vi "Verify Can Add Additional Bitfile.vi"(8 "error in (no error)":errorcluster, 10 "RIO Device Addresses":string[](array[string]), 11 "Item Ref in":T1 format="%.0x") -> (0 "error out":errorcluster, 2 "Can Add?":bool, 3 "Item Ref out":T1 format="%.0x")   [LabVIEW 2015, in "Engine Simulation Toolkit System Explorer.lvlib"]
uses:
  Engine Simulation Toolkit System Explorer.lvlib
  <vilib>/NI Veristand/Custom Device API/Custom Device Item Ref.ctl
  Shared/Bitfile EST Version.ctl
  Shared/Properties.vi
  <vilib>/NI Veristand/Custom Device API/Get Item Property (String).vi
  Shared/Engine Simulation Toolkit Shared.lvlib
  <vilib>/NI VeriStand/Custom Device API/Custom Device API.lvlib
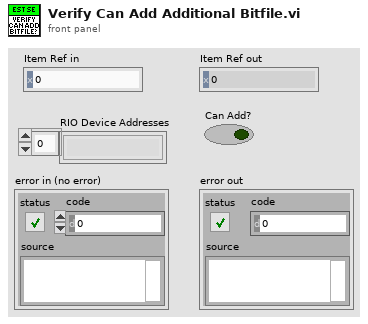
[diagram p1: front panel]
types:
  T1 = typedef "Custom Device API.lvlib/Custom Device Item Ref.ctl" = u64
  T2 = typedef "Engine Simulation Toolkit Shared.lvlib/Bitfile EST Version.ctl" = enum16{"1.0", "1.1", "1.2", "1.3", "1.4"}
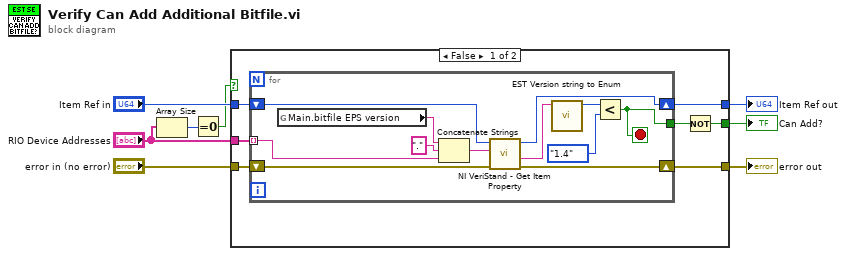
[diagram p0: block diagram]
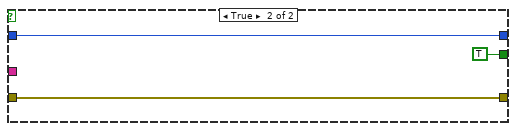
[diagram p2: hidden frame]
diagram:
  n1 = Array Size(array="RIO Device Addresses") -> (size(s)=w2:i32)
  n2 = Equal To 0?(x=w2) -> (x = 0?=w1:bool)
  n3 = case shown="False" w1 {
    tunnel: [w14 w28] -> w8
    tunnel: "Item Ref in" -> [w13 w28]
    tunnel: [w12 w29] -> w6
    tunnel: "error in (no error)" -> [w11 w29]
    tunnel: [w10 TRUE] -> w4
    tunnel: "RIO Device Addresses" -> [w9 _]
    frame False {
      n4 = for {
        tunnel: w9 -> [w25] mode=indexing
        shift-right: [w23] -> w12
        shift-left: w11 -> [w24]
        shift-right: [w20] -> w14
        shift-left: w13 -> [w21]
        tunnel: [w16] -> w15
        stop <- w16 stop-if-true
        n5 = global read "Properties.vi" "Main.bitfile EPS version"() -> (w27:string)
        n6 = Concatenate Strings(w27, "." ("string"), w25) -> (w22:string)
        n7 = call-poly <vilib>:"NI VeriStand - Get Item Property.vi"("error in (no error)"=w24, "Property Name"=w22, "Item Ref in"=w21) -> ("error out"=w23:errorcluster, "Value"=w19:string, "Item Ref out"=w20:T1)  [unwired: 5 in, 1 out]
        n8 = call "EST Version string to Enum.vi"("EST version string"=w19) -> ("EST version enum"=w18:T2)  [unwired: 9 in, 1 out]
        n9 = Less?(x=w18, y=Bitfile_EST_Version."1.4") -> (x < y?=w16:bool)
      }
      n10 = Not(x=w15) -> (.not. x?=w10:bool)
    }
    frame True {
    }
  }
  "Can Add?" <- w4
  "Item Ref out" <- w8
  "error out" <- w6
